vi "fgt get sensor Calibration.vi"(8 "error in (no error)":errorcluster, 11 "sensorIndex":u32) -> (0 "error out":errorcluster, 3 "calibration out":T1=enum."H2O")   [LabVIEW 2016, in "fgt_SDK.lvlib"]
doc: "Get internal used calibration table by the sensor."
uses:
  fgt_SDK.lvlib
  TypeDefs/fgt_SENSOR_CALIBRATION.ctl
  dlls/fgt_SDK_32.dll
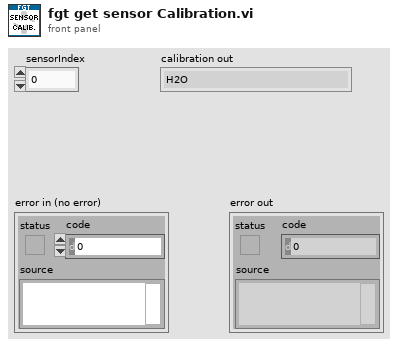
[diagram p1: front panel]
types:
  T1 = typedef "fgt_SDK.lvlib/fgt_SENSOR_CALIBRATION.ctl" = enum16{"None", "H2O", "IPA", "HFE", "FC40", "OIL"}
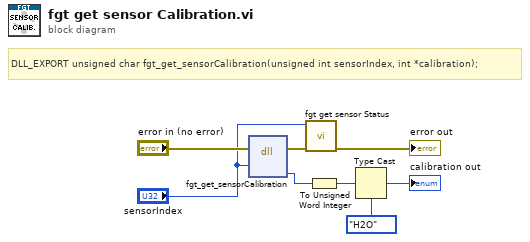
[diagram p0: block diagram]
diagram:
  # "DLL_EXPORT unsigned char fgt_get_sensorCalibration(unsigned int sensorIndex, int *calibration);"
  n1 = dll-call lib="PTH2Zabs D\nMes DocumentsDéveloppementFluigentSDKsfgt-sdk-labviewdllsfgt_SDK_*.*" fn="fgt_get_sensorCalibration"(error in="error in (no error)", "sensorIndex"="sensorIndex") -> (error out=w7:errorcluster, "calibration"=w4:i32)  [unwired: 5 in, 1 out]
  n2 = call "fgt get sensor Status.vi"("error in (no error)"=w7, "pressureIndex"="sensorIndex") -> ("error out"=→"error out":errorcluster)  [unwired: 9 in]
  n3 = To Unsigned Word Integer(number=w4) -> (unsigned 16bit integer=w3:u16)
  n4 = Type Cast(type=fgt_SENSOR_CALIBRATION."H2O" ("calibration out"), x=w3) -> (*(type *) &x=→"calibration out":T1)
